vi "Read Image Format.vi"(8 "error in (no error)":errorcluster, 11 "MSOX6004 in":refnum<class "MSOX6004.lvclass">) -> (0 "error out":errorcluster, 2 "Image Format":T1, 3 "MSOX6004 out":refnum<class "MSOX6004.lvclass">)   [LabVIEW 2018, in "MSOX6004.lvlib" / "MSOX6004.lvclass"]
uses:
  MSOX6004.lvclass
  Custom Controls/Image Format.ctl
  MSOX6004.lvclass/MSOX6004.ctl
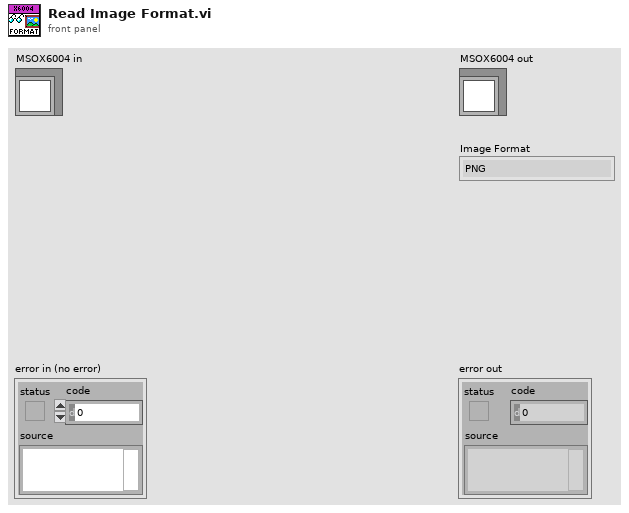
[diagram p1: front panel]
types:
  T1 = typedef "MSOX6004.lvlib/MSOX6004.lvclass/Image Format.ctl" = enum16{"PNG", "BMP"}
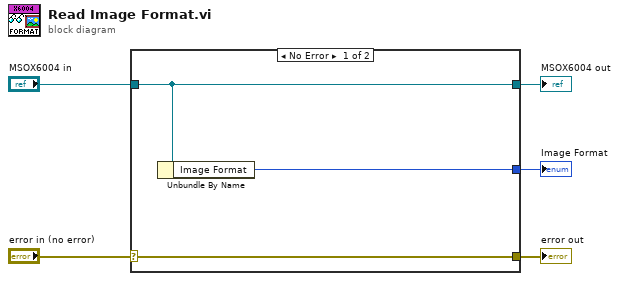
[diagram p0: block diagram]
diagram:
  n1 = case shown="No Error" "error in (no error)" {
    selector: "error in (no error)" -> [w8 w9]
    tunnel: [w8 w9] -> w4
    tunnel: [w7 w10] -> w2
    tunnel: "MSOX6004 in" -> [w7 w10]
    tunnel: [w6 _] -> w1
    frame No Error {
      n2 = Unbundle By Name(w7) -> ("Image Format"=w6:T1)
    }
    frame Error {
    }
  }
  "error out" <- w4
  "MSOX6004 out" <- w2
  "Image Format" <- w1
